vi "VI Server_Get Menu Ring Item Names.vi"(7 "Label":string, 8 "error in":errorcluster, 11 "VI Server Cluster":T1) -> (0 "error out":errorcluster, 1 "Control Reference":refnum<vi>, 2 "Item Names (String[])":string[](array[string]), 3 "VI Server Cluster.DUP":T1, 4 "Value":u16, 6 "Label.Text":string caption="Label.Text DUP")   [LabVIEW 2020, in "VI Server Toolkit LV2013.lvlib"]
doc: "Returns item names (STR array) of the Menu Ring."
uses:
  VI Server Toolkit LV2013.lvlib
  VI Server_TypeDefs/VI Server_RefsCluster.ctl
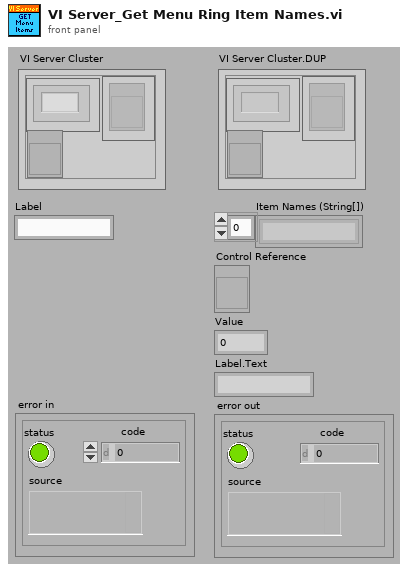
[diagram p1: front panel]
types:
  T1 = typedef "VI Server_RefsCluster.ctl" = cluster{"Labels":string[], "Refs":refnum<vi>[], "VI Ref":refnum<vi>}
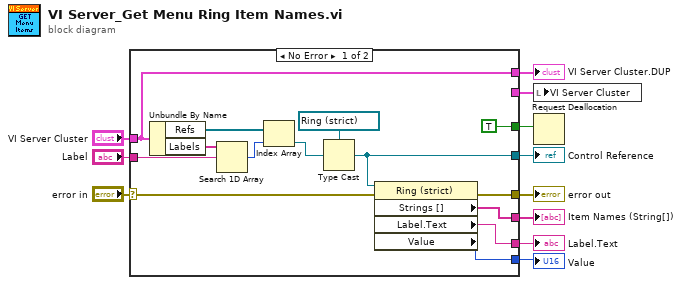
[diagram p0: block diagram]
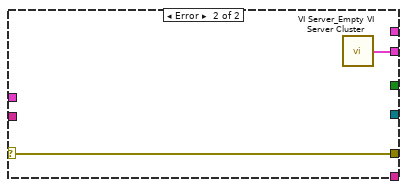
[diagram p2: hidden frame]
diagram:
  n1 = case shown="No Error" "error in" {
    selector: "error in" -> [w20 w27]
    tunnel: "Label" -> [w24 _]
    tunnel: "VI Server Cluster" -> [w16 _]
    tunnel: [w19 w27] -> w11
    tunnel: [w18 _] -> w7
    tunnel: [w17 _] -> w6
    tunnel: [w16 _] -> w5
    tunnel: [w15 _] -> w4
    tunnel: [w14 _] -> w3
    tunnel: [TRUE _] -> w2
    tunnel: [_ w26] -> w1
    frame No Error {
      n2 = Unbundle By Name(w16) -> ("Refs"=w22:refnum<vi>[], "Labels"=w25:string[])
      n3 = Search 1D Array(1D array=w25, element=w24) -> (index of element=w23:i32)  [unwired: 1 out]
      n4 = Index Array(array=w22, index=w23) -> (element=w21:refnum<vi>)
      n5 = Type Cast(type=refnum<vi> refnum ("Ring"), x=w21) -> (*(type *) &x=w18:refnum<vi>)
      n6 = property class="Ring (strict)"(reference=w18, error in=w20) -> (error out=w19:errorcluster, "Strings []"=w15:string[], "Label.Text"=w17:string, "Value"=w14:u16)  [unwired: 1 out]
    }
    frame Error {
      n7 = call "VI Server_Empty VI Server Cluster.vi"() -> ("VI Server Cluster"=w26:T1)  [unwired: 7 in]
    }
  }
  "error out" <- w11
  "VI Server Cluster.DUP" <- w5
  "Control Reference" <- w7
  "Label.Text" <- w6
  "Item Names (String[])" <- w4
  "Value" <- w3
  n8 = local write "VI Server Cluster"(w1) -> ()
  n9 = Request Deallocation(w2) -> ()
